vi "M05 Hydraulic cells.vi"(11 "EV3 in":T1) -> (3 "EV3 out":T1)   [LabVIEW 2016]
uses:
  <vilib>/NXT/Subs/LVHSConnector.ctl
  <vilib>/NXT/LegoClasses/BrickReference/BrickReference.lvclass
  <vilib>/NXT/Dual Mode Library/Waits/Wait_Num.vi
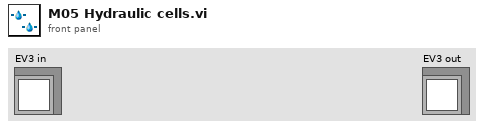
[diagram p1: front panel]
types:
  T1 = typedef "LVHSConnector.ctl" = refnum<class "BrickReference.lvclass">
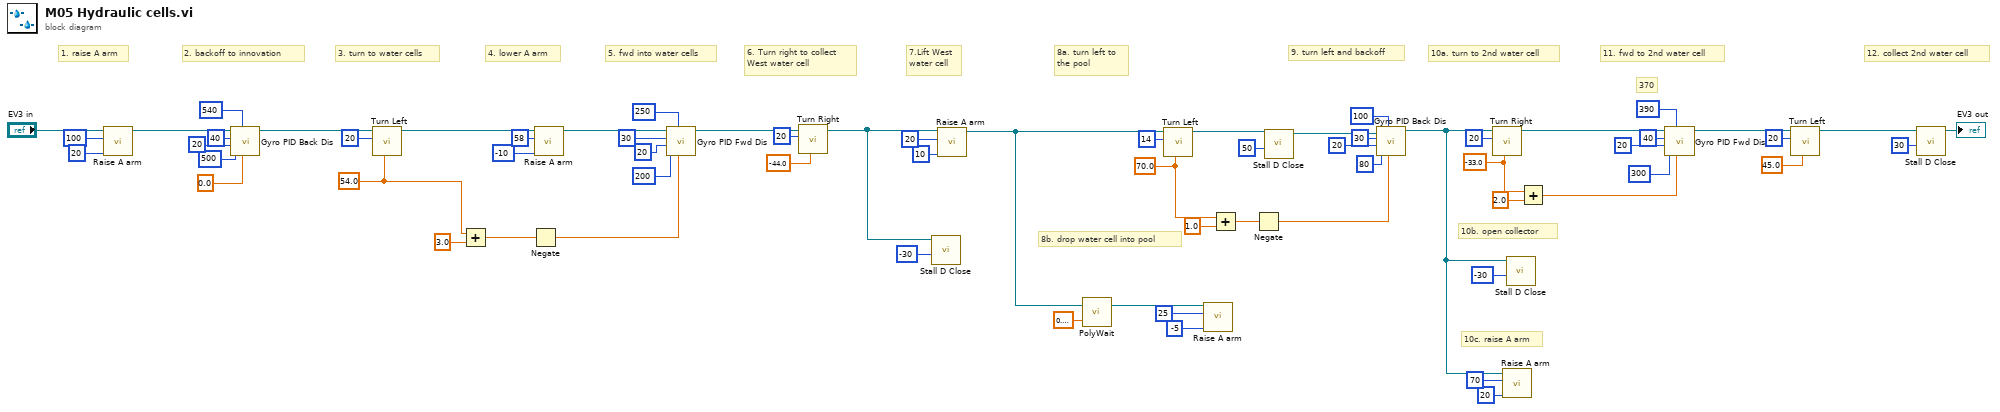
[diagram p0: block diagram]
diagram:
  w15 = sgl -33.0 ("Turning angle")
  w18 = sgl 70.0 ("Turning angle")
  w47 = sgl 54.0 ("Turning angle")
  # "370"
  # "12. collect 2nd water cell"
  # "11. fwd to 2nd water cell"
  # "10c. raise A arm"
  # "10b. open collector"
  # "10a. turn to 2nd water cell"
  # "9. turn left and backoff"
  # "8b. drop water cell into pool"
  # "8a. turn left to\nthe pool"
  # "7.Lift West\nwater cell"
  # "6. Turn right to collect\nWest water cell"
  # "5. fwd into water cells"
  # "4. lower A arm"
  # "3. turn to water cells"
  # "2. backoff to innovation"
  # "1. raise A arm"
  n1 = call "Raise A arm.vi"("Power"=i8 20, "Rotation"=100, "EV3 in"="EV3 in") -> ("EV3 out"=w63:T1)  [unwired: 8 in]
  n2 = call "Gyro PID Back Dis.vi"("Target angle"=sgl 0.0, "Threshold to stop"=540 ("Threshold to Color"), "Threshold to slow"=500, "Min. speed"=20, "Max. speed"=40, "EV3 in"=w63) -> ("EV3 out"=w57:T1)  [unwired: 5 in]
  n3 = call "Turn Left.vi"("Turning angle"=w47, "Motor B (right)"=i8 20, "EV3 in"=w57) -> ("EV3 out"=w50:T1)  [unwired: 8 in]
  n4 = Add(x=w47, y=sgl 3.0) -> (x+y=w45:sgl)
  n5 = Negate(x=w45) -> (-x=w44:sgl)
  n6 = call "Raise A arm.vi"("Power"=i8 -10, "Rotation"=58, "EV3 in"=w50) -> ("EV3 out"=w48:T1)  [unwired: 8 in]
  n7 = call "Gyro PID Fwd Dis.vi"("Target angle"=w44, "Threshold to stop"=250, "Threshold to slow"=200, "Min. speed"=20, "Max. speed"=30, "EV3 in"=w48) -> ("EV3 out"=w43:T1)  [unwired: 5 in]
  n8 = call "Turn Right.vi"("Turning angle"=sgl -44.0, "Motor B (right)"=i8 20, "EV3 in"=w43) -> ("EV3 out"=w9:T1)  [unwired: 8 in]
  n9 = call "Stall D Close.vi"("Power"=i8 -30, "NXT/EV3"=w9) -> ()  [unwired: 9 in, 1 out]
  n10 = call "Raise A arm.vi"("Power"=i8 10, "Rotation"=20, "EV3 in"=w9) -> ("EV3 out"=w7:T1)  [unwired: 8 in]
  n11 = call-poly <vilib>:"PolyWait.vi"("Time (1 sec)"=sgl 0.6, "NXT/EV3"=w7) -> ("NXT/EV3"=w12:T1)  [unwired: 2 in]
  n12 = call "Turn Left.vi"("Turning angle"=w18, "Motor B (right)"=i8 14, "EV3 in"=w7) -> ("EV3 out"=w6:T1)  [unwired: 8 in]
  n13 = call "Raise A arm.vi"("Power"=i8 -5, "Rotation"=25, "EV3 in"=w12) -> ()  [unwired: 8 in, 1 out]
  n14 = Add(x=w18, y=sgl 1.0) -> (x+y=w17:sgl)
  n15 = Negate(x=w17) -> (-x=w4:sgl)
  n16 = call "Stall D Close.vi"("Power"=i8 50, "NXT/EV3"=w6) -> ("NXT/EV3"=w5:T1)  [unwired: 9 in]
  n17 = call "Gyro PID Back Dis.vi"("Target angle"=w4, "Threshold to stop"=100, "Threshold to slow"=80, "Min. speed"=20, "Max. speed"=30, "EV3 in"=w5) -> ("EV3 out"=w22:T1)  [unwired: 5 in]
  n18 = call "Turn Right.vi"("Turning angle"=w15, "Motor B (right)"=i8 20, "EV3 in"=w22) -> ("EV3 out"=w26:T1)  [unwired: 8 in]
  n19 = call "Raise A arm.vi"("Power"=i8 20, "Rotation"=70, "EV3 in"=w22) -> ()  [unwired: 8 in, 1 out]
  n20 = call "Stall D Close.vi"("Power"=i8 -30, "NXT/EV3"=w22) -> ()  [unwired: 9 in, 1 out]
  n21 = Add(x=w15, y=sgl 2.0) -> (x+y=w14:sgl)
  n22 = call "Gyro PID Fwd Dis.vi"("Target angle"=w14, "Threshold to stop"=390, "Threshold to slow"=300, "Min. speed"=20, "Max. speed"=40, "EV3 in"=w26) -> ("EV3 out"=w21:T1)  [unwired: 5 in]
  n23 = call "Turn Left.vi"("Turning angle"=sgl 45.0, "Motor B (right)"=i8 20, "EV3 in"=w21) -> ("EV3 out"=w3:T1)  [unwired: 8 in]
  n24 = call "Stall D Close.vi"("Power"=i8 30, "NXT/EV3"=w3) -> ("NXT/EV3"=→"EV3 out":T1)  [unwired: 9 in]
